vi "readLUT.vi"(8 "error in (no error)":errorcluster, 11 "AOTF in":refnum<class "AOTF.lvclass">) -> (0 "error out":errorcluster, 3 "AOTF out":refnum<class "AOTF.lvclass">)   [LabVIEW 2012, in "AOTF.lvclass"]
uses:
  AOTF.lvclass
  Controls/MaxPower cluster.ctl
  Controls/LUT cluster.ctl
  AOTF.lvclass/AOTF.ctl
  <vilib>/Utility/file.llb/Read From Spreadsheet File (DBL).vi
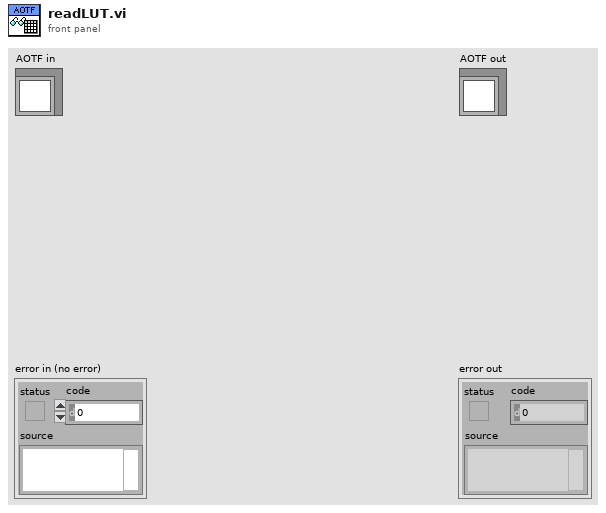
[diagram p1: front panel]
types:
  T1 = typedef "LUT cluster.ctl" = cluster{"LUT Array":dbl[][][]}
  T2 = typedef "MaxPower cluster.ctl" = cluster{"MaxPower Array":dbl[]}
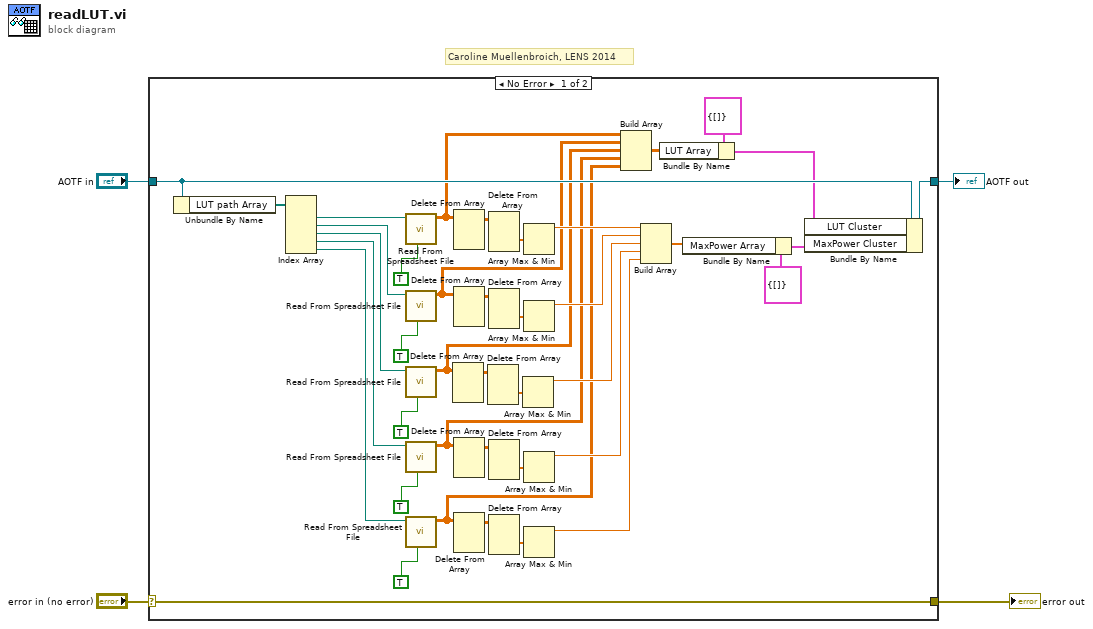
[diagram p0: block diagram]
diagram:
  # "Caroline Muellenbroich, LENS 2014"
  n1 = case shown="No Error" "error in (no error)" {
    selector: "error in (no error)" -> [w44 w46]
    tunnel: [w44 w46] -> w3
    tunnel: [w41 w45] -> w1
    tunnel: "AOTF in" -> [w42 w45]
    frame No Error {
      n2 = Unbundle By Name(w42) -> ("LUT path Array"=w38:path[])
      n3 = Index Array(array=w38) -> (element #1=w37:path, element #2=w24:path, element #3=w23:path, element #4=w22:path, element #5=w21:path)  [unwired: 5 in]
      n4 = call-poly <vilib>:"Read From Spreadsheet File.vi"("transpose (no:F)"=TRUE, "file path (dialog if empty)"=w37) -> ("all rows"=w12:dbl[][])  [unwired: 5 in, 4 out]
      n5 = call-poly <vilib>:"Read From Spreadsheet File.vi"("transpose (no:F)"=TRUE, "file path (dialog if empty)"=w24) -> ("all rows"=w11:dbl[][])  [unwired: 5 in, 4 out]
      n6 = call-poly <vilib>:"Read From Spreadsheet File.vi"("transpose (no:F)"=TRUE, "file path (dialog if empty)"=w23) -> ("all rows"=w8:dbl[][])  [unwired: 5 in, 4 out]
      n7 = call-poly <vilib>:"Read From Spreadsheet File.vi"("transpose (no:F)"=TRUE, "file path (dialog if empty)"=w22) -> ("all rows"=w7:dbl[][])  [unwired: 5 in, 4 out]
      n8 = call-poly <vilib>:"Read From Spreadsheet File.vi"("transpose (no:F)"=TRUE, "file path (dialog if empty)"=w21) -> ("all rows"=w6:dbl[][])  [unwired: 5 in, 4 out]
      n9 = Delete From Array(array=w8) -> (array with subset deleted=w29:dbl[][])  [unwired: 3 in, 1 out]
      n10 = Delete From Array(array=w12) -> (array with subset deleted=w40:dbl[][])  [unwired: 3 in, 1 out]
      n11 = Delete From Array(array=w11) -> (array with subset deleted=w32:dbl[][])  [unwired: 3 in, 1 out]
      n12 = Delete From Array(array=w7) -> (array with subset deleted=w35:dbl[][])  [unwired: 3 in, 1 out]
      n13 = Delete From Array(array=w6) -> (array with subset deleted=w26:dbl[][])  [unwired: 3 in, 1 out]
      n14 = Delete From Array(array=w29) -> (deleted portion=w30:dbl[])  [unwired: 3 in, 1 out]
      n15 = Delete From Array(array=w40) -> (deleted portion=w39:dbl[])  [unwired: 3 in, 1 out]
      n16 = Delete From Array(array=w32) -> (deleted portion=w31:dbl[])  [unwired: 3 in, 1 out]
      n17 = Delete From Array(array=w35) -> (deleted portion=w36:dbl[])  [unwired: 3 in, 1 out]
      n18 = Delete From Array(array=w26) -> (deleted portion=w25:dbl[])  [unwired: 3 in, 1 out]
      n19 = Array Max & Min(array=w30) -> (max value=w18:dbl)  [unwired: 3 out]
      n20 = Array Max & Min(array=w39) -> (max value=w20:dbl)  [unwired: 3 out]
      n21 = Array Max & Min(array=w31) -> (max value=w19:dbl)  [unwired: 3 out]
      n22 = Array Max & Min(array=w36) -> (max value=w17:dbl)  [unwired: 3 out]
      n23 = Array Max & Min(array=w25) -> (max value=w16:dbl)  [unwired: 3 out]
      n24 = Build Array(w12, w11, w8, w7, w6) -> (w10:dbl[][][])
      n25 = Build Array(w20, w19, w18, w17, w16) -> (w15:dbl[])
      n26 = Bundle By Name(cluster=T1 {"LUT Array"=[]} ("LUT Cluster"), "LUT Array"=w10) -> (w9:T1)
      n27 = Bundle By Name(cluster=T2 {"MaxPower Array"=[]} ("MaxPower Cluster"), "MaxPower Array"=w15) -> (w13:T2)
      n28 = Bundle By Name(cluster=w42, "LUT Cluster"=w9, "MaxPower Cluster"=w13) -> (w41:refnum<class "AOTF.lvclass">)
    }
    frame Error {
    }
  }
  "error out" <- w3
  "AOTF out" <- w1
